vi "CreatePublicEvents.vi"(8 "error in (no error)":errorcluster, 11 "SMO.UI":refnum<class "SMO.UI.lvclass">) -> (0 "error out":errorcluster, 3 "SMO.UI out":refnum<class "SMO.UI.lvclass">)   [LabVIEW 2013, in "SMO.UI.lvclass"]
uses:
  SMO.UI.lvclass
  SMO/SMO.lvclass
  SMO.UI.lvclass/SMO.UI.ctl
panel:
  # "For instructions on how to use the JKI State Machine Objects, examples and video tutorials, visit:\nhttp://jki.net/state-machine-objects/\n\nJKI State Machine Objects™\nhttp://jki.net/state-machine-objects/\nCopyright (C) 2005-2015, JKI <info@jki.net>\nALL RIGHTS RESERVED"
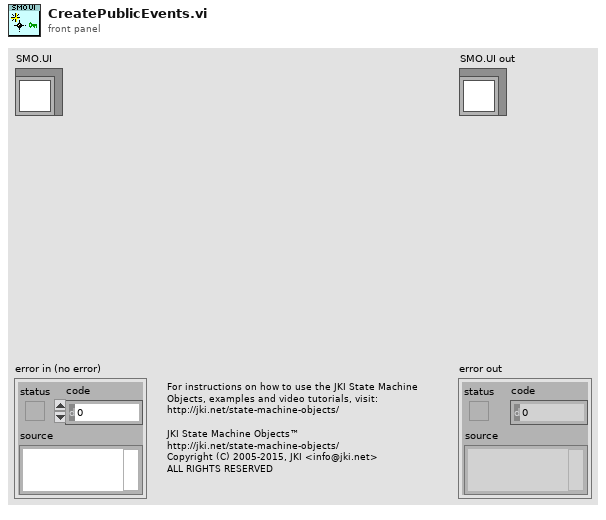
[diagram p1: front panel]
types:
  T1 = typedef "SMO.UI.lvclass/PrivateData--Ref.ctl" = refnum<data-value>
  T2 = typedef "SMO.UI.lvclass/PrivateData--Cluster.ctl" = cluster{"Public Events":T3, "Private Events":T4}
  T3 = typedef "SMO.UI.lvclass/PublicEvents--Cluster.ctl" = cluster{"UI Hidden":refnum<user-event>}
  T4 = typedef "SMO.UI.lvclass/PrivateEvents--Cluster.ctl" = cluster{"Show-Hide UI":refnum<user-event>}
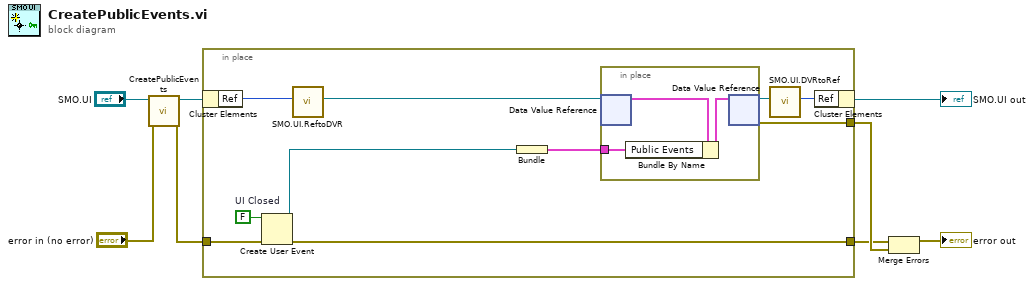
[diagram p0: block diagram]
diagram:
  n1 = call-parent "CreatePublicEvents.vi"("error in (no error)"="error in (no error)", "SMO"="SMO.UI") -> ("error out"=w2:errorcluster, "SMO out"=w3:refnum<class "SMO.UI.lvclass">)  [unwired: 8 in]
  n2 = in-place {
    in-place-border: [w18] -> w8
    in-place-border: w2 -> [w14]
    in-place-border: [w12] -> w1
    w15 = FALSE  # UI Closed
    n3 = in-place-cluster #1(w3) -> ("Ref"=w17:u32)
    n4 = Create User Event(user event datatype=w15, error in=w14) -> (user event=w9:refnum<user-event>, error out=w12:errorcluster)
    n5 = call "SMO.UI.ReftoDVR.vi"("Ref"=w17) -> ("Ref"=w16:T1)  [unwired: 10 in]
    n6 = Bundle("UI Closed"=w9) -> (w13:cluster{"UI Closed":refnum<user-event>})  [unwired: 1 in]
    n7 = in-place {
      in-place-border: w13 -> [w19]
      n8 = in-place-dvr #2(w16) -> (w21:T2)  [unwired: 1 out]
      n9 = Bundle By Name(cluster=w21, "Public Events"=w19) -> (w20:T2)
      n10 = in-place-dvr #2(w20) -> (w11:T1, w18:errorcluster)
    }
    n11 = call "SMO.UI.DVRtoRef.vi"("Ref"=w11) -> ("Ref"=w10:u32)  [unwired: 10 in]
    n12 = in-place-cluster #1("Ref"=w10) -> (→"SMO.UI out":refnum<class "SMO.UI.lvclass">)
  }
  n13 = Merge Errors(w1, w8) -> (→"error out":errorcluster)
